vi "AB_Update_Version_Info.vi"(8 "error in (no error)":errorcluster, 10 "Build spec name":string, 11 "TargetFile in":refnum<class "AB_Targetfile.lvclass">) -> (0 "error out":errorcluster, 3 "TargetFile out":refnum<class "AB_Targetfile.lvclass">)   [LabVIEW 2020]
uses:
  <vilib>/AppBuilder/AB_Classes/TargetFile/AB_Targetfile.lvclass
  e:/builds/penguin/labview/branches/2020/dev/dist/vi.lib/AppBuilder/AB_Classes/Build/AB_Build.lvclass
  <vilib>/AppBuilder/AB_Classes/Build/AB_Build.lvclass
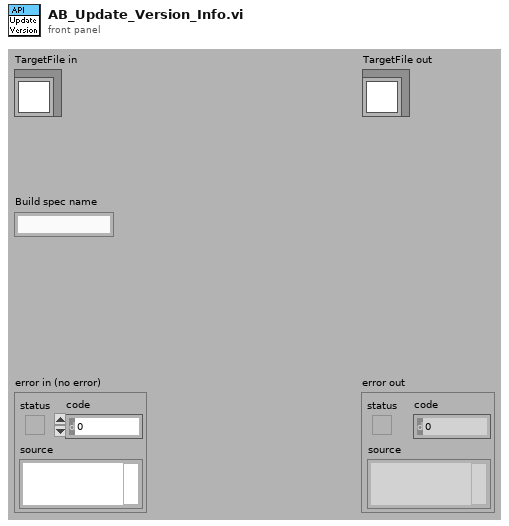
[diagram p1: front panel]
types:
  T1 = typedef "AB_Targetfile.ctl" = cluster{"targetfileName":string, "targetfileGUID":string, "enableDebugging":bool, "versionInfo":cluster{"productName":string, "legalCopyright":string, "companyName":string, "internalName":string, "fileDescription":string}, "eng_consolidatedTypeInfo":string, "fastFileFormat":bool, "eng_LEIFBuildData":u32, "versionIndependent":bool}
  T2 = typedef "AB_Build.ctl" = cluster{"buildSpecName":string, "buildSpecDescription":string, "destinations":refnum<class "AB_Destination.lvclass">[], "exclusionOption":T3, "defaultLanguage":string, "supportedLanguages":string[], "excludedDirectories":path[], "buildContext":refnum<vi>, "buildObject":T4, "preview":bool, "programatic":bool, "progressBarEvents":T5, "userLog_Path":path, "preActionID":string, "preAction_Path":path, "postActionID":string, "postAction_Path":path, "eng_checkForBrokenVIs?":bool, "eng_verboseLinkerErrors?":bool, "localDest_Path":path, "targetDest_Path":path, "removeVIObject":u16, "cache":refnum<class "PreviewCache.lvclass">, "use cache":bool, "previewCache_ID":string, "buildCache_ID":string, "eng_TempLocalDest_Path":path, "eng_collectDependencies?":bool, "versionInfo":cluster{"buildVersion":cluster{"major":u16, "minor":u16, "patch":u16, "build":u16}, "autoIncrement":bool}, "eng_enableVIChecksums":bool}
  T3 = typedef "AB_Exclusion_Option.ctl" = cluster{"typedefs":bool, "polymorphicVIs":bool, "unusedLibraryItems":bool, "modifyLibraryFile":bool, "edit-timeDependencies":bool, "inlineVIs":bool, "dependent PPLs":bool, "dependent DLLs":bool}
  T4 = typedef "ItemRef.ctl" = u64
  T5 = typedef "provcom_ProgressBar_Events.ctl" = cluster{"newJob":refnum<user-event>, "newItem":refnum<user-event>, "errorMsg":T6, "cancel":refnum<user-event>}
  T6 = typedef "mxLvBuildError.ctl" = refnum<user-event>
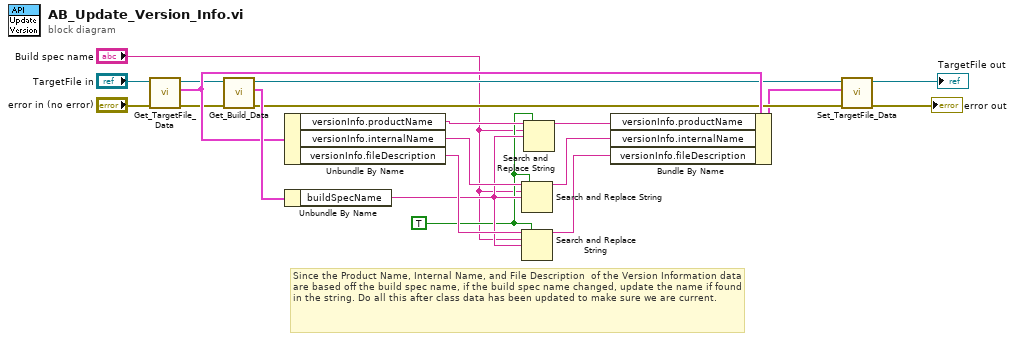
[diagram p0: block diagram]
diagram:
  w11 = TRUE ("replace all? (F)")
  # "Since the Product Name, Internal Name, and File Description  of the Version Information data are based off the build spec name, if the build spec name changed, update the name if found in the string. Do all this after class data has been updated to make sure we are current."
  n1 = call <vilib>:"Get_TargetFile_Data.vi"("error in (no error)"="error in (no error)", "AB_Targetfile in"="TargetFile in") -> ("error out"=w6:errorcluster, "data"=w10:T1, "AB_Targetfile out"=w5:refnum<class "AB_Targetfile.lvclass">)  [unwired: 7 in]
  n2 = call <vilib>:"Get_Build_Data.vi"("error in (no error)"=w6, "Class in"=w5) -> ("error out"=w9:errorcluster, "data"=w19:T2, "Class out"=w4:refnum<class "AB_Targetfile.lvclass">)  [unwired: 7 out]
  n3 = Unbundle By Name(w10) -> ("versionInfo.productName"=w18:string, "versionInfo.internalName"=w16:string, "versionInfo.fileDescription"=w14:string)
  n4 = Unbundle By Name(w19) -> ("buildSpecName"=w13:string)
  n5 = Search and Replace String(replace all?=w11, input string=w16, search string="Build spec name", replace string=w13) -> (result string=w15:string)  [unwired: 1 in, 6 out]
  n6 = Search and Replace String(replace all?=w11, input string=w14, search string="Build spec name", replace string=w13) -> (result string=w12:string)  [unwired: 1 in, 6 out]
  n7 = Search and Replace String(replace all?=w11, input string=w18, search string="Build spec name", replace string=w13) -> (result string=w17:string)  [unwired: 2 in, 5 out]
  n8 = Bundle By Name(cluster=w10, "versionInfo.productName"=w17, "versionInfo.internalName"=w15, "versionInfo.fileDescription"=w12) -> (w1:T1)
  n9 = call <vilib>:"Set_TargetFile_Data.vi"("error in (no error)"=w9, "data"=w1, "AB_Targetfile in"=w4) -> ("error out"=→"error out":errorcluster, "AB_Targetfile out"=→"TargetFile out":refnum<class "AB_Targetfile.lvclass">)  [unwired: 7 in]
